vi "request.vi"(0 "Device In":T1, 3 "error in":errorcluster) -> (7 "Device Out":T1, 8 "Comm":T2, 10 "error out":errorcluster)   [LabVIEW 2019]
uses:
  <userlib>/IoT Devices/_subVIs/HTTPComm.ctl
  <vilib>/httpClient/POSTBuffer.vi
  <vilib>/httpClient/LabVIEWHTTPClient.lvlib
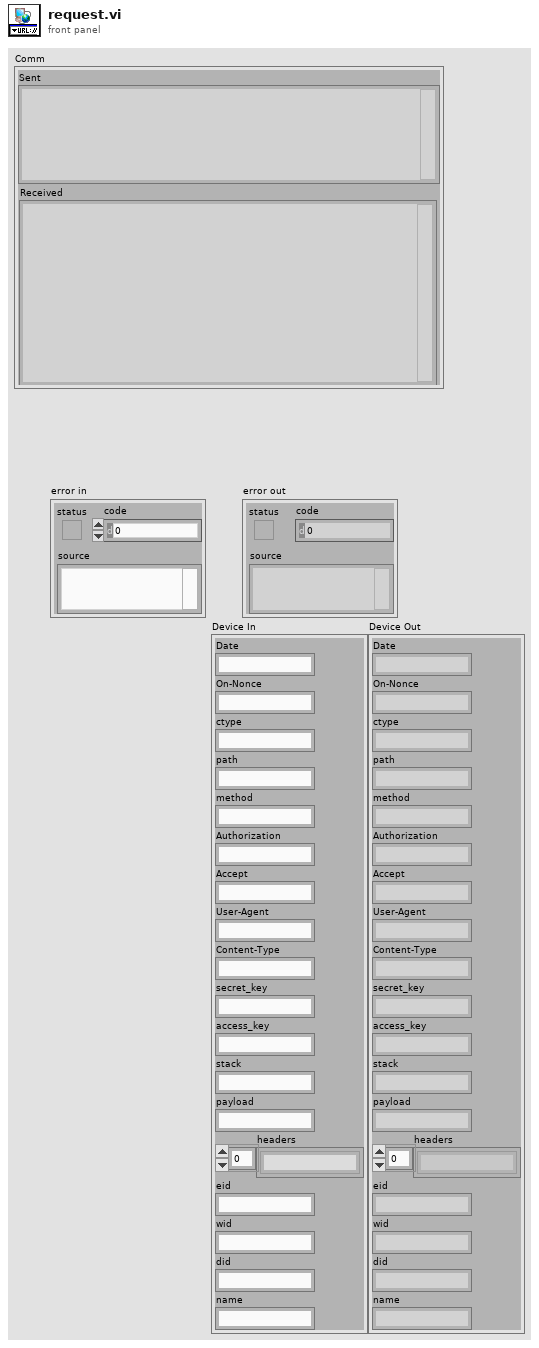
[diagram p1: front panel]
types:
  T1 = cluster{"Date":string, "On-Nonce":string, "ctype":string, "path":string, "method":string, "Authorization":string, "Accept":string, "User-Agent":string, "Content-Type":string, "secret_key":string, "access_key":string, "stack":string, "payload":string, "headers":string[], "eid":string, "wid":string, "did":string, "name":string}
  T2 = typedef "HTTPComm.ctl" = cluster{"url":string, "sent headers":string, "sent body":string, "headers":string, "body":string, "Sent":string, "Received":string}
  T3 = typedef "LabVIEWHTTPClient.lvlib/ClientHandle.ctl" = refnum<k1>
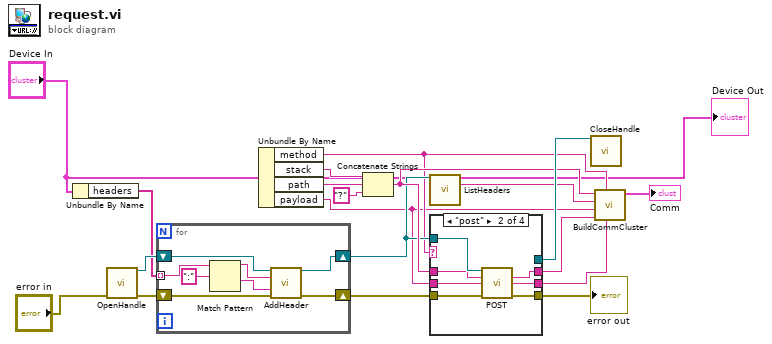
[diagram p0: block diagram]
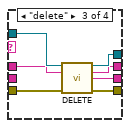
[diagram p3: hidden frame]
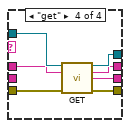
[diagram p4: hidden frame]
diagram:
  n1 = Unbundle By Name("Device In") -> ("headers"=w17:string[])
  n2 = call <vilib>:"OpenHandle.vi"("error in (no error)"="error in") -> ("client handle out"=w18:T3, "error out"=w16:errorcluster)  [unwired: 13 in]
  n3 = for {
    shift-right: [w26] -> w8
    shift-left: w18 -> [w27]
    shift-right: [w24] -> w15
    shift-left: w16 -> [w25]
    tunnel: w17 -> [w20] mode=indexing
    n4 = Match Pattern(string=w20, regular expression=":") -> (before substring=w22:string, after substring=w21:string)  [unwired: 1 in, 2 out]
    n5 = call <vilib>:"AddHeader.vi"("client handle"=w27, "header"=w22, "value"=w21, "error in (no error)"=w25) -> ("client handle out"=w26:T3, "error out"=w24:errorcluster)  [unwired: 10 in]
  }
  n6 = Unbundle By Name("Device In") -> ("method"=w4:string, "stack"=w12:string, "path"=w11:string, "payload"=w3:string)
  n7 = Concatenate Strings(w12, w11, "?") -> (w9:string)
  n8 = call <vilib>:"ListHeaders.vi"("client handle"=w8) -> ("headers"=w7:string)  [unwired: 12 in, 2 out]
  n9 = case shown="\"post\"" w4 {
    tunnel: w8 -> [_ w35 w42 w49]
    tunnel: [_ _ w41 w48] -> w19
    tunnel: [_ w34 w39 w46] -> w5
    tunnel: [_ w33 w40 w47] -> w6
    tunnel: w15 -> [w28 w32 w38 w45]
    tunnel: [w28 w31 w37 w44] -> w14
    tunnel: w9 -> [_ w30 w36 w43]
    tunnel: w3 -> [_ w29 _ _]
    frame "False", Default {
    }
    frame "post" {
      n10 = call-poly <vilib>:"POST.vi"("client handle"=w35, "url"=w30, "buffer"=w29, "error in (no error)"=w32) -> ("headers"=w33:string, "body"=w34:string, "error out"=w31:errorcluster)  [unwired: 8 in, 1 out]
    }
    frame "delete" {
      n11 = call <vilib>:"DELETE.vi"("client handle"=w42, "url"=w36, "error in (no error)"=w38) -> ("client handle out"=w41:T3, "headers"=w40:string, "body"=w39:string, "error out"=w37:errorcluster)  [unwired: 9 in]
    }
    frame "get" {
      n12 = call <vilib>:"GET.vi"("client handle"=w49, "url"=w43, "error in (no error)"=w45) -> ("client handle out"=w48:T3, "headers"=w47:string, "body"=w46:string, "error out"=w44:errorcluster)  [unwired: 9 in]
    }
  }
  "error out" <- w14
  n13 = call <vilib>:"CloseHandle.vi"("client handle"=w19) -> ()  [unwired: 14 in, 1 out]
  n14 = call "BuildCommCluster.vi"("reply body"=w5, "Type"=w4, "reply headers"=w6, "sent body"=w3, "sent headers"=w7, "url"=w9) -> ("Comm"=→"Comm":T2)  [unwired: 5 in]
  "Device Out" <- "Device In"
